vi "Read target point.vi"(8 "error in (no error)":errorcluster, 11 "Target Point in":refnum<class "Target Point.lvclass">) -> (0 "error out":errorcluster, 2 "target point":cluster{"x":i16, "y":i16}, 3 "Target Point out":refnum<class "Target Point.lvclass">)   [LabVIEW 2014, in "Target Point.lvclass"]
uses:
  Target Point.lvclass
  Target Point.lvclass/Target Point.ctl
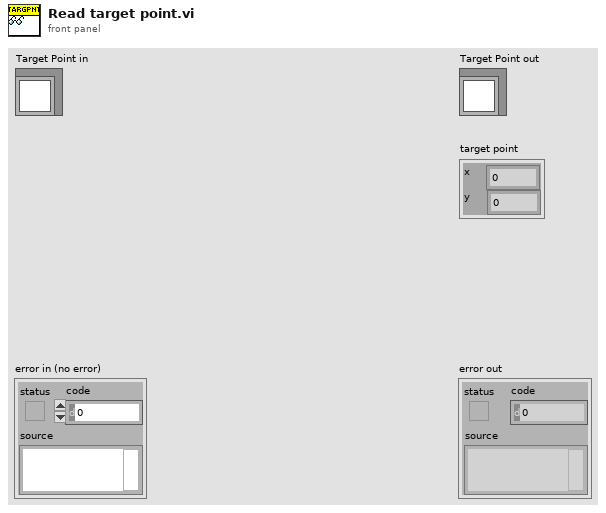
[diagram p1: front panel]
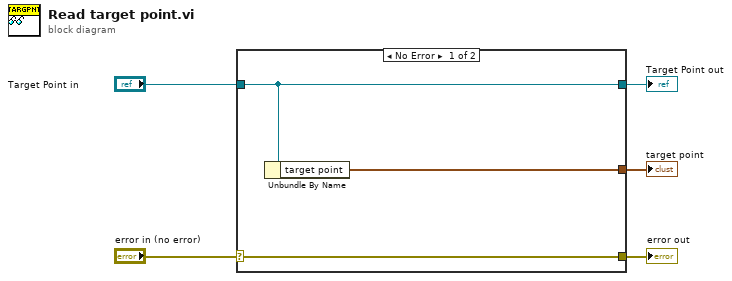
[diagram p0: block diagram]
diagram:
  n1 = case shown="No Error" "error in (no error)" {
    selector: "error in (no error)" -> [w8 w9]
    tunnel: [w8 w9] -> w4
    tunnel: [w7 w10] -> w2
    tunnel: "Target Point in" -> [w7 w10]
    tunnel: [w6 _] -> w1
    frame No Error {
      n2 = Unbundle By Name(w7) -> ("target point"=w6:cluster{"x":i16, "y":i16})
    }
    frame Error {
    }
  }
  "error out" <- w4
  "Target Point out" <- w2
  "target point" <- w1
